vi "Read TagName.vi"(11 "Proccess in":refnum<class "Proccess.lvclass">) -> (2 "TagName":string)   [LabVIEW 2019, in "Proccess.lvclass"]
uses:
  Proccess.lvclass
  Proccess.lvclass/Proccess.ctl
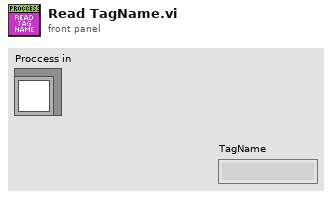
[diagram p1: front panel]
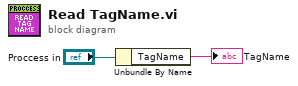
[diagram p0: block diagram]
diagram:
  n1 = Unbundle By Name("Proccess in") -> ("TagName"=→"TagName":string)
